vi "LCD Example.vi"() -> ()   [LabVIEW 2013]
doc: "This example shows how to use the NI Vision seven-segment display reader VIs to read values that are displayed on a LCD panel."
uses:
  <vilib>/vision/NI_Vision_Development_Module.lvlib
panel:
  out "Image":T1(plugin-control)
  out "Segments status":T2(array[cluster])
  in  "Delay":i32(slide)=738 max=3000 scale=0.0..1000.0
  out "Output value":i32
  in  "stop":bool
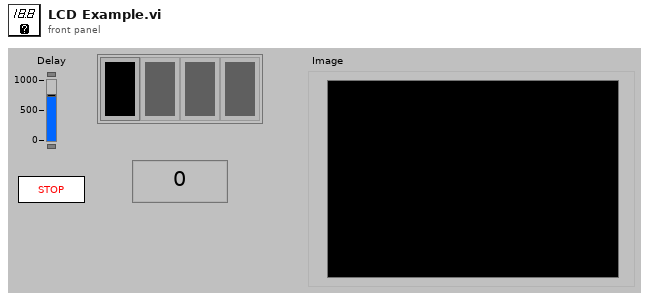
[diagram p1: front panel]
types:
  T1 = typedef "IMAQ Image.ctl" = refnum<image>
  T2 = cluster{bool, bool, bool, bool, bool, bool, bool}[]
  T3 = cluster{i32[], cluster{"Contour Type":u32, "ROI Type":u32, i32[]}[]}
  T4 = cluster{"Global Rectangle":i32[], "Contours":cluster{"ID":enum32{"External", "Internal"}, "Type":u32, "Coordinates":i32[]}[]}
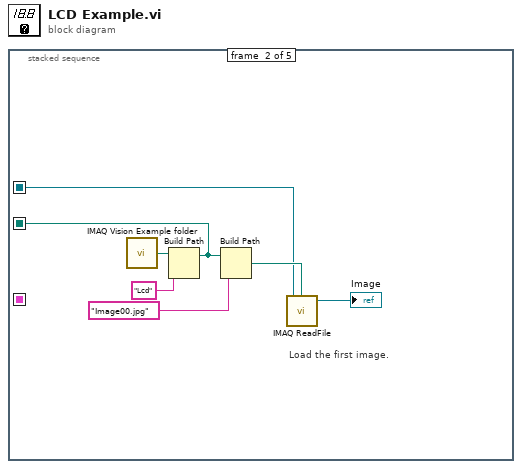
[diagram p0: block diagram]
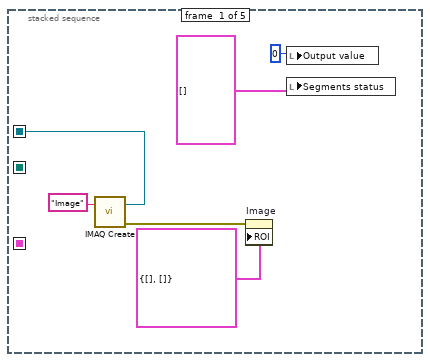
[diagram p2: hidden frame]
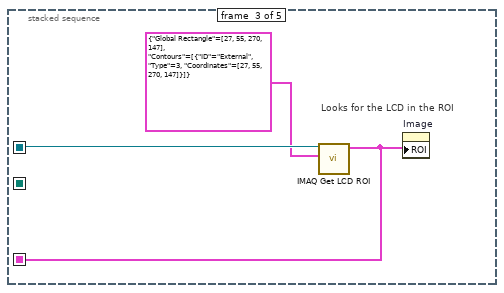
[diagram p3: hidden frame]
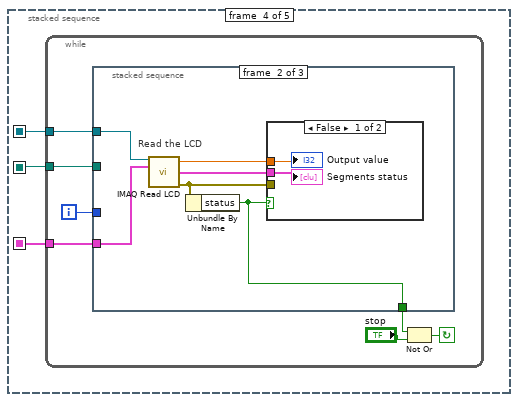
[diagram p4: hidden frame]
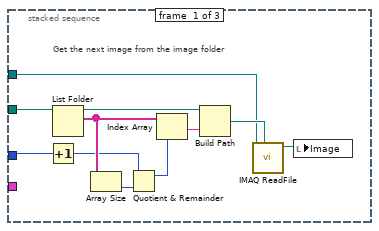
[diagram p5: hidden frame]
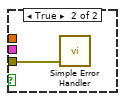
[diagram p6: hidden frame]
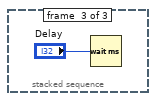
[diagram p7: hidden frame]
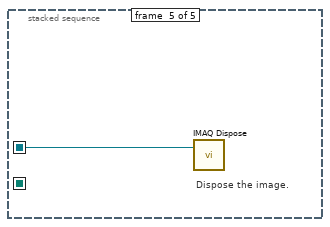
[diagram p8: hidden frame]
diagram:
  n1 = stacked-sequence {
    seq-local: [w5 _ _ _ _] -> [_ w9 w16 w18 w48]
    seq-local: [_ _ w15 _ _] -> [_ _ _ w19 _]
    seq-local: [_ w10 _ _ _] -> [_ _ _ w17 _]
    frame #0 {
      n2 = call "IMAQ Create"("Image Name"="Image") -> ("New Image"=w5:T1, "error out"=w2:errorcluster)  [unwired: 3 in, 1 out]
      n3 = property on="Image" class="ImageControl"(error in=w2, "ROI"=T3 {[], []}) -> ()  [unwired: 1 in, 2 out]
      n4 = local write "Output value"(0 ("Output value")) -> ()
      n5 = local write "Segments status"(T2 [] ("Segments status")) -> ()
    }
    frame #1 {
      # "Load the first image."
      n6 = call "IMAQ Vision Example folder.vi"() -> ("Example Image Path"=w7:path)  [unwired: 1 in]
      n7 = Build Path(base path=w7, name or relative path="Lcd") -> (appended path=w10:path)
      n8 = Build Path(base path=w10, name or relative path="Image00.jpg") -> (appended path=w11:path)
      n9 = call "IMAQ ReadFile"("File Path"=w11, "Image"=w9) -> ("Image Out"=→"Image":T1)  [unwired: 3 in, 6 out]
    }
    frame #2 {
      # "Looks for the LCD in the ROI"
      n10 = call "IMAQ Get LCD ROI"("ROI Descriptor"=T4 {"Global Rectangle"=[27, 55, 270, 147], "Contours"=[{"ID"=enum."External", "Type"=3, "Coordinates"=[27, 55, 270, 147]}]}, "Image"=w16) -> ("ROI Descriptor out"=w15:T4)  [unwired: 3 in, 6 out]
      n11 = property on="Image" class="ImageControl"("ROI"=w15) -> ()  [unwired: 2 in, 2 out]
    }
    frame #3 {
      n12 = while {
        tunnel: w17 -> [w21]
        tunnel: w18 -> [w23]
        tunnel: w19 -> [w25]
        i -> [w22]
        stop <- w24 continue-if-true
        n13 = stacked-sequence {
          tunnel: w25 -> [_ w43 _]
          tunnel: w23 -> [w30 w40 _]
          tunnel: w22 -> [w29 _ _]
          tunnel: w21 -> [w28 _ _]
          tunnel: [_ w39 _] -> w20
          frame #0 {
            # "Get the next image from the image folder"
            n14 = Increment(x=w29) -> (x+1=w31:i32)
            n15 = List Folder(path=w28) -> (path out=w33:path, filenames=w37:string[])  [unwired: 1 in, 4 out]
            n16 = Array Size(array=w37) -> (size(s)=w36:i32)
            n17 = Quotient & Remainder(x=w31, y=w36) -> (x-y*floor(x/y)=w35:i32)  [unwired: 1 out]
            n18 = Index Array(array=w37, index=w35) -> (element=w34:string)
            n19 = Build Path(base path=w33, name or relative path=w34) -> (appended path=w32:path)
            n20 = call "IMAQ ReadFile"("File Path"=w32, "Image"=w30) -> ("Image Out"=w27:T1)  [unwired: 3 in, 6 out]
            n21 = local write "Image"(w27) -> ()
          }
          frame #1 {
            # "Read the LCD"
            n22 = call "IMAQ Read LCD"("Image"=w40, "ROI Descriptor"=w43) -> ("Output value"=w42:dbl, "Segments status"=w41:T2, "error out"=w38:errorcluster)  [unwired: 5 in, 6 out]
            n23 = Unbundle By Name(w38) -> ("status"=w39:bool)
            n24 = case shown="False" w39 {
              tunnel: w42 -> [w45 _]
              tunnel: w41 -> [w44 _]
              tunnel: w38 -> [_ w46]
              frame False {
                "Output value" <- w45
                "Segments status" <- w44
              }
              frame True {
                n25 = call <vilib>:"Simple Error Handler.vi"("error in (no error)"=w46) -> ()  [unwired: 1 in, 8 out]
              }
            }
          }
          frame #2 {
            n26 = Wait (ms)(milliseconds to wait="Delay") -> ()  [unwired: 1 out]
          }
        }
        n27 = Not Or(1:"stop", 2:w20) -> (0:w24:bool)
      }
    }
    frame #4 {
      # "Dispose the image."
      n28 = call "IMAQ Dispose"("Image"=w48) -> ()  [unwired: 2 in, 4 out]
    }
  }
